vi "Launch.vi"(8 "error in (no error)":errorcluster, 10 "Run":bool, 11 "Binary Instr in":refnum<class "Binary Instr.lvclass">) -> (0 "error out":errorcluster, 3 "Binary Instr out":refnum<class "Binary Instr.lvclass">)   [LabVIEW 2015, in "Item Actor.lvlib" / "Binary Instr.lvclass"]
uses:
  Binary Instr.lvclass
  Instrument Information/Instrument.lvclass/Instrument.ctl
  Instrument Information/Read App Path.vi
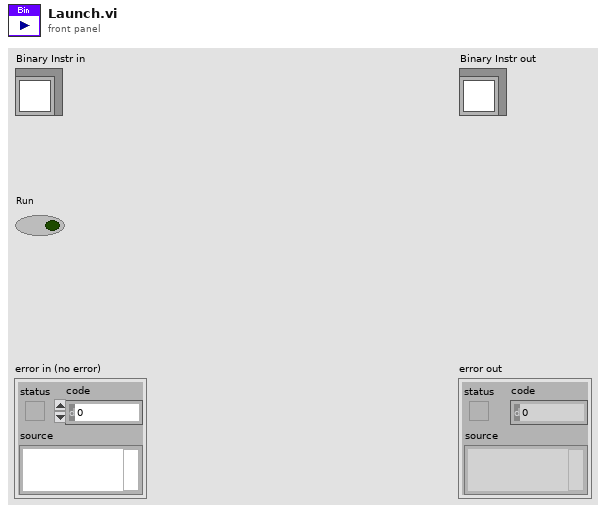
[diagram p1: front panel]
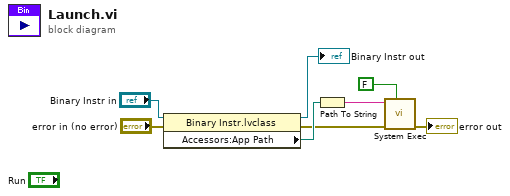
[diagram p0: block diagram]
diagram:
  n1 = property class="Binary Instr.lvclass"(reference="Binary Instr in", error in="error in (no error)") -> (reference out=→"Binary Instr out":refnum<class "Binary Instr.lvclass">, error out=w4:errorcluster, "Accessors:App Path"=w6:path)
  n2 = Path To String(path=w6) -> (string=w5:string)
  n3 = call <vilib>:"System Exec.vi"("wait until completion? (T)"=FALSE, "error in (no error)"=w4, "command line"=w5) -> ("error out"=→"error out":errorcluster)  [unwired: 5 in, 3 out]
